vi "LJStreamUD get and check exp config.vi"(0 "Working Directory In":path, 1 "App Name":string) -> (4 "Write To File":bool, 6 "Data File Prefix":string="data", 7 "Interval (ms)":u32=500, 9 "Resolution":u8, 10 "Graph History":i32=1000 min=0, 11 "SettlingFactor":u8, 13 "Device Config File Name":string, 14 "# Channels":i32=4, 16 "Disable Scaling":bool, 17 "Max File Size (Bytes)":i32=1048576, 18 "Channel Setup":T1={"+Ch"=["0", "1", "2", "3", "4", "5", "6", "7"], "-Ch"=["199", "199", "199", "199", "199", "199", "199", "199"], "Ranges"=[0, 0, 0, 0, 0, 0, 0, 0], "Scaling Equation"=["y=v0", "y=v1", "y=v2", "y=v3", "y=v4", "y=v5", "y=v6", "y=v7"], "Graph?"=[]} {"Ranges" items=["LJ_rgBIP10V", "LJ_rgBIP5V", "LJ_rgUNI5V", "LJ_rgUNI2P5V", "LJ_rgUNI1P25V", "LJ_rgBIP1V", "LJ_rgUNIP625V", "LJ_rgBIPP1V", "LJ_rgBIPP01V"]}, 19 "error out":errorcluster)   [LabVIEW 2020]
panel:
  out "Scan Rate (Hz)":dbl=500.0 format="%.3f"
  out "Device Config Path":path
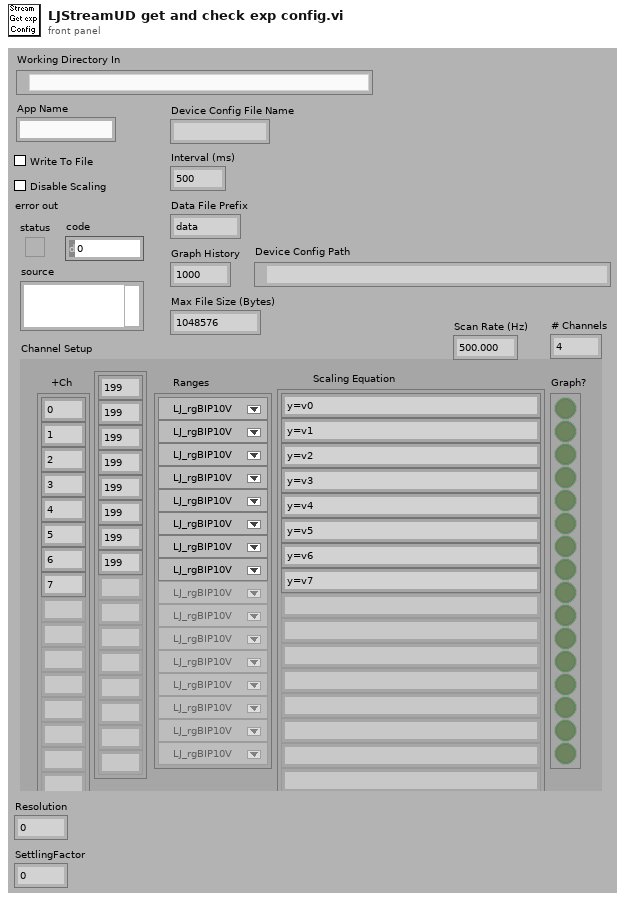
[diagram p1: front panel]
types:
  T1 = cluster{"+Ch":string[], "-Ch":string[], "Ranges":u16[], "Scaling Equation":string[], "Graph?":bool[]}
  T2 = enum16{"Left Button", "Center Button", "Right Button", "Window Close"}
  T3 = enum32{"existing file", "new file", "new or existing file", "existing dir", "new dir", "new or existing dir", "existing file (use LLBs)", "new file (use LLBs)", "new or existing file (use LLBs)", "new or existing file or directory (use LLBs)"}
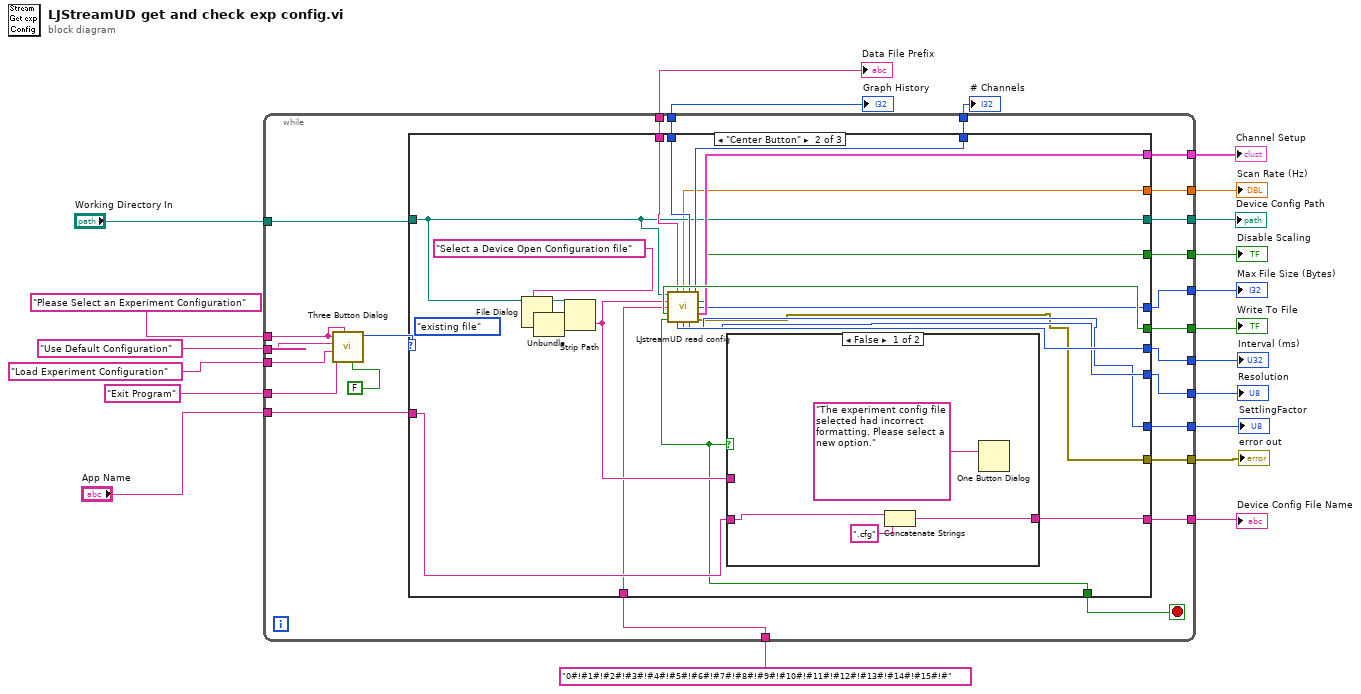
[diagram p0: block diagram]
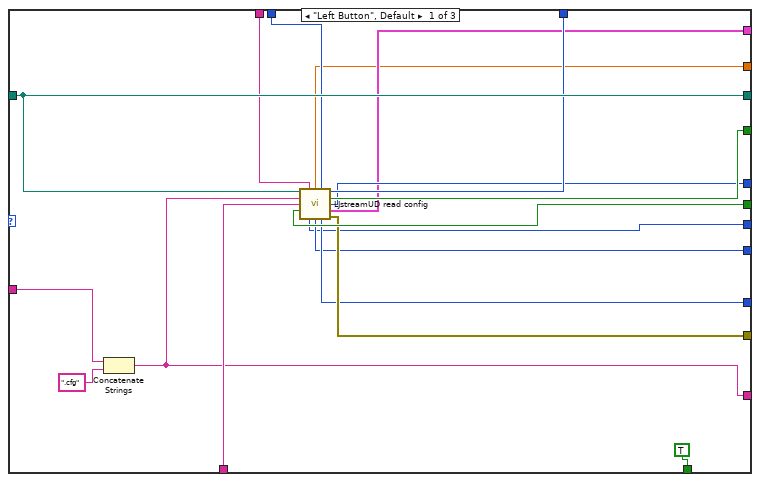
[diagram p2: hidden frame]
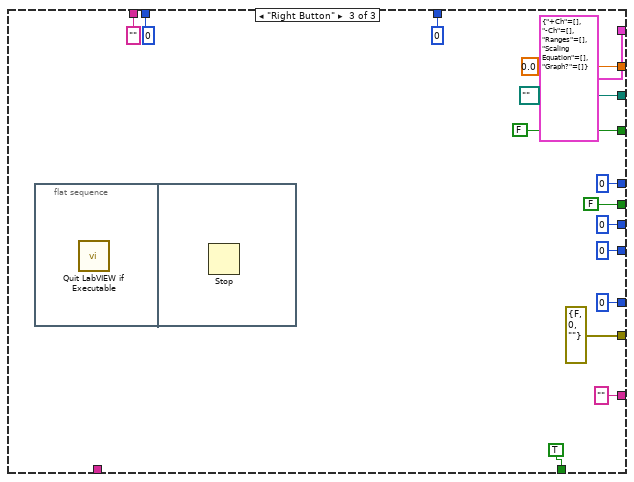
[diagram p4: hidden frame]
diagram:
  n1 = while {
    tunnel: "Working Directory In" -> [w45]
    tunnel: "App Name" -> [w44]
    tunnel: [w43] -> w19
    tunnel: "Use Default Configuration" ("F button name (\"Cancel\")") -> [w26]
    tunnel: "Load Experiment Configuration" ("T button name (\"OK\")") -> [w25]
    tunnel: "Please Select an Experiment Configuration" ("message") -> [w27]
    tunnel: [w41] -> w15
    tunnel: [w40] -> w14
    tunnel: [w39] -> w13
    tunnel: [w38] -> w12
    tunnel: [w37] -> w11
    tunnel: [w36] -> w10
    tunnel: [w35] -> w9
    tunnel: [w34] -> w8
    tunnel: [w33] -> w7
    tunnel: [w32] -> w6
    tunnel: [w31] -> w5
    tunnel: [w30] -> w4
    tunnel: [w29] -> w3
    tunnel: "Exit Program" ("Right Button Text (\"Cancel\")") -> [w24]
    tunnel: "0#!#1#!#2#!#3#!#4#!#5#!#6#!#7#!#8#!#9#!#10#!#11#!#12#!#13#!#14#!#15#!#" ("ChP Default") -> [w22]
    stop <- w23 stop-if-true
    n2 = call <vilib>:"Three Button Dialog.vi"("Allow user to close window? (TRUE)"=FALSE, "Window Title (\"\")"=w27, "Right Button Text (\"Cancel\")"=w24, "Center Button Text (\"No\")"=w25, "Left Button Text (\"Yes\")"=w26, "message"=w27) -> ("Which Button?"=w42:T2)  [unwired: 5 in]
    n3 = case shown="\"Center Button\"" w42 {
      tunnel: w45 -> [w58 w70 _]
      tunnel: w44 -> [w62 w82 _]
      tunnel: [w58 w70 path "" ("Working Directory In")] -> w43
      tunnel: [w61 w80 FALSE ("Write To File")] -> w41
      tunnel: [w48 w79 u32 0 ("Interval (ms)")] -> w40
      tunnel: [w57 w71 "" ("Data File Prefix")] -> w39
      tunnel: [w56 w72 0 ("Graph History")] -> w38
      tunnel: [w55 w73 0 ("# Channels")] -> w37
      tunnel: [w54 w74 FALSE ("Disable Scaling")] -> w36
      tunnel: [w53 w75 0 ("Max File Size (Bytes)")] -> w35
      tunnel: [w52 w76 T1 {"+Ch"=[], "-Ch"=[], "Ranges"=[], "Scaling Equation"=[], "Graph?"=[]} ("Channel Setup")] -> w34
      tunnel: w22 -> [w60 w68 _]
      tunnel: [w59 w81 "" ("name")] -> w33
      tunnel: [w51 w67 errorcluster {"status"=FALSE, "code"=0, "source"=""} ("error out")] -> w32
      tunnel: [w49 w78 u8 0 ("Resolution")] -> w31
      tunnel: [w50 w77 u8 0 ("SettlingFactor")] -> w30
      tunnel: [w47 w66 0.0 ("Scan Rate (Hz)")] -> w29
      tunnel: [TRUE ("Good Config") w65 TRUE ("Good Config")] -> w23
      frame "Left Button", Default {
        n4 = Concatenate Strings(w62, ".cfg" ("filename")) -> (w59:string)
        n5 = call "LJstreamUD read config.vi"("Working Directory"=w58, "filename"=w59, "ChP Default"=w60) -> ("Data File Prefix"=w57:string, "Scan Rate (Hz)"=w47:dbl, "Graph History"=w56:i32, "# Channels"=w55:i32, "Disable Scaling"=w54:bool, "Max File Size (Bytes)"=w53:i32, "Write To File"=w61:bool, "Channel Setup"=w52:T1, "Interval (ms)"=w48:u32, "Resolution"=w49:u8, "SettlingFactor"=w50:u8, "error out"=w51:errorcluster)  [unwired: 1 out]
      }
      frame "Center Button" {
        (unwired) T3."existing file" ("select mode (2)")
        n6 = File Dialog(7:"Select a Device Open Configuration file" ("Substring"), 11:w70) -> (0:w64:errorcluster, 3:w83:path)  [unwired: 5 in, 2 out]
        n7 = Unbundle(w64) -> ()  [unwired: 3 out]
        n8 = Strip Path(path=w83) -> (name=w69:string)  [unwired: 1 out]
        n9 = call "LJstreamUD read config.vi"("Working Directory"=w70, "filename"=w69, "ChP Default"=w68) -> ("Data File Prefix"=w71:string, "Scan Rate (Hz)"=w66:dbl, "Graph History"=w72:i32, "# Channels"=w73:i32, "Disable Scaling"=w74:bool, "Max File Size (Bytes)"=w75:i32, "Write To File"=w80:bool, "Channel Setup"=w76:T1, "Good Config"=w65:bool, "Interval (ms)"=w79:u32, "Resolution"=w78:u8, "SettlingFactor"=w77:u8, "error out"=w67:errorcluster)
        n10 = case shown="False" w65 {
          tunnel: w82 -> [w86 _]
          tunnel: [w85 w89] -> w81
          tunnel: w69 -> [_ w89]
          frame False {
            n11 = Concatenate Strings(w86, ".cfg" ("string")) -> (w85:string)
            n12 = One Button Dialog(message="The experiment config file selected had incorrect formatting. Please select a new option.") -> ()  [unwired: 1 in, 1 out]
          }
          frame True {
          }
        }
      }
      frame "Right Button" {
        n13 = flat-sequence {
          frame #0 {
            n14 = call "Quit LabVIEW if Executable.vi"() -> ()  [unwired: 1 in]
          }
          frame #1 {
            n15 = Stop() -> ()  [unwired: 1 in]
          }
        }
      }
    }
  }
  "Device Config Path" <- w19
  "Device Config File Name" <- w7
  "error out" <- w6
  "Interval (ms)" <- w14
  "Write To File" <- w15
  "Data File Prefix" <- w13
  "Graph History" <- w12
  "# Channels" <- w11
  "Disable Scaling" <- w10
  "Max File Size (Bytes)" <- w9
  "Channel Setup" <- w8
  "Scan Rate (Hz)" <- w3
  "Resolution" <- w5
  "SettlingFactor" <- w4
